vi "HISW-GetVIpath.vi"(8 "error in (no error)":errorcluster, 11 "HISW in":refnum<class "HISW.lvclass">) -> (0 "error out":errorcluster, 2 "MethodsPath":path, 3 "HISW out":refnum<class "HISW.lvclass">)   [LabVIEW 2020, in "HISW.lvclass"]
doc: "Get the path of the HISW methods"
uses:
  HISW.lvclass
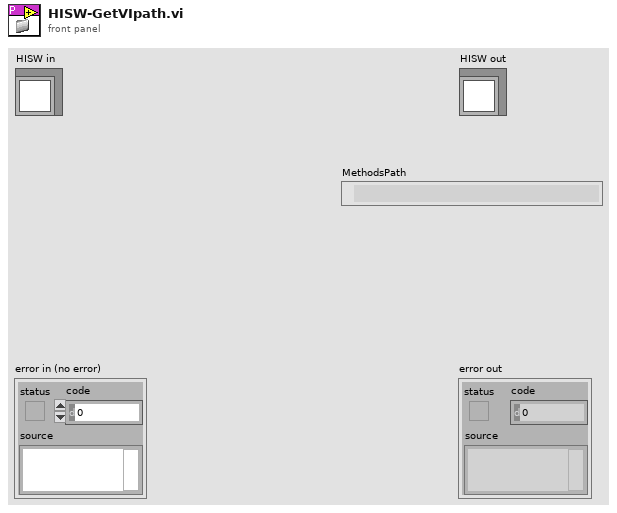
[diagram p1: front panel]
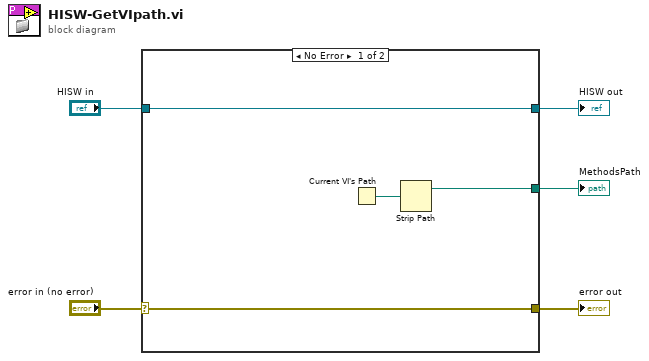
[diagram p0: block diagram]
diagram:
  n1 = case shown="No Error" "error in (no error)" {
    selector: "error in (no error)" -> [w8 w11]
    tunnel: [w8 w11] -> w4
    tunnel: [w9 w10] -> w2
    tunnel: "HISW in" -> [w9 w10]
    tunnel: [w6 _] -> w1
    frame No Error {
      n2 = Current VI's Path() -> (path=w7:path)
      n3 = Strip Path(path=w7) -> (stripped path=w6:path)  [unwired: 1 out]
    }
    frame Error {
    }
  }
  "error out" <- w4
  "HISW out" <- w2
  "MethodsPath" <- w1
